vi "MergeFileAutoConfigMARLIN.vi"(4 "error in (no error)":errorcluster, 6 "test num":u32, 7 "ProjetIN":string) -> (0 "error out":errorcluster, 2 "MergeFileConfigOUT":T1, 3 "ProjetOUT":string)   [LabVIEW 2017]
uses:
  DefDeType/MergeFileConfig.ctl
  DefDeType/WhichPath.ctl
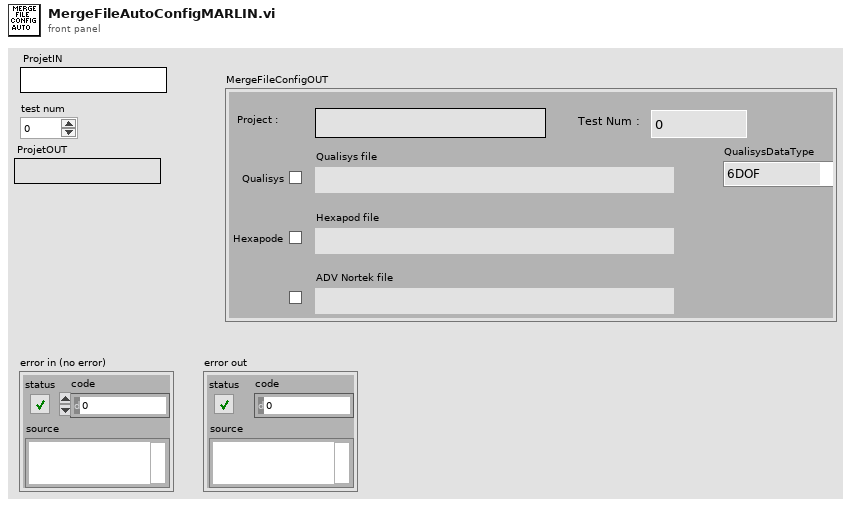
[diagram p1: front panel]
types:
  T1 = typedef "MergeFileConfig.ctl" = cluster{"Test Num : ":u32, "Project :":string, "Qualisys file":path, "Hexapod file":path, "ADV Nortek file":path, "QualisysDataType":enum16{"6DOF", "3DTracking", "6DOF + 3D"}, "Qualisys":bool, "Hexapode":bool, "ADV Nortek":bool}
  T2 = typedef "WhichPath.ctl" = enum16{"DossierProjet", "Config", "Meas", "MeasSuitCase", "MeasOnBoard", "MeasQualisys", "MeasTDMS", "MeasHexapode", "MeasNortek", "Fig", "Res", "MeasUSB"}
  T3 = typedef "WhichPath.ctl" = enum16{"DossierProjet", "Config", "Meas", "MeasPCI", "MeasCRIO1", "MeasCRIO2", "MeasQualisys", "MeasHBM", "MeasTDMS", "Fig", "Res"}
  T4 = typedef "ConfigTotale.ctl" = cluster{"VoltageChannels":T5, "WheastoneBridgeChannels":T6, "Configuration":T7}
  T5 = typedef "VoltageChannels.ctl" = cluster{"ChannelNames":string[], "Sensitivity(Unit/V)":dbl[], "AutoZero":bool[], "ChannelUnits":string[], "Offsets(Units)":dbl[], "Graph Num":u8[]}
  T6 = typedef "WBridgeChannels.ctl" = cluster{"ChannelNames":string[], "Sensitivity(Unit/V)":dbl[], "AutoZero":bool[], "ChannelUnits":string[], "Offsets(Units)":dbl[], "Graph Num":u8[]}
  T7 = typedef "Configuration.ctl" = cluster{"AcqSamplingRate(Hz)":u32, "AcqTime(s)":u32, "Trigger":bool, "NbVoltageChannels":u32, "NbWBridgeChannels":u32, "Qualisys":bool, "Hexapode":bool, "FinalSamplingRate(Hz)":u32, "QualisysDataType":enum16{"6DOF", "3DTracking", "6DOF + 3D"}, "Nortek":bool, "HBM":bool}
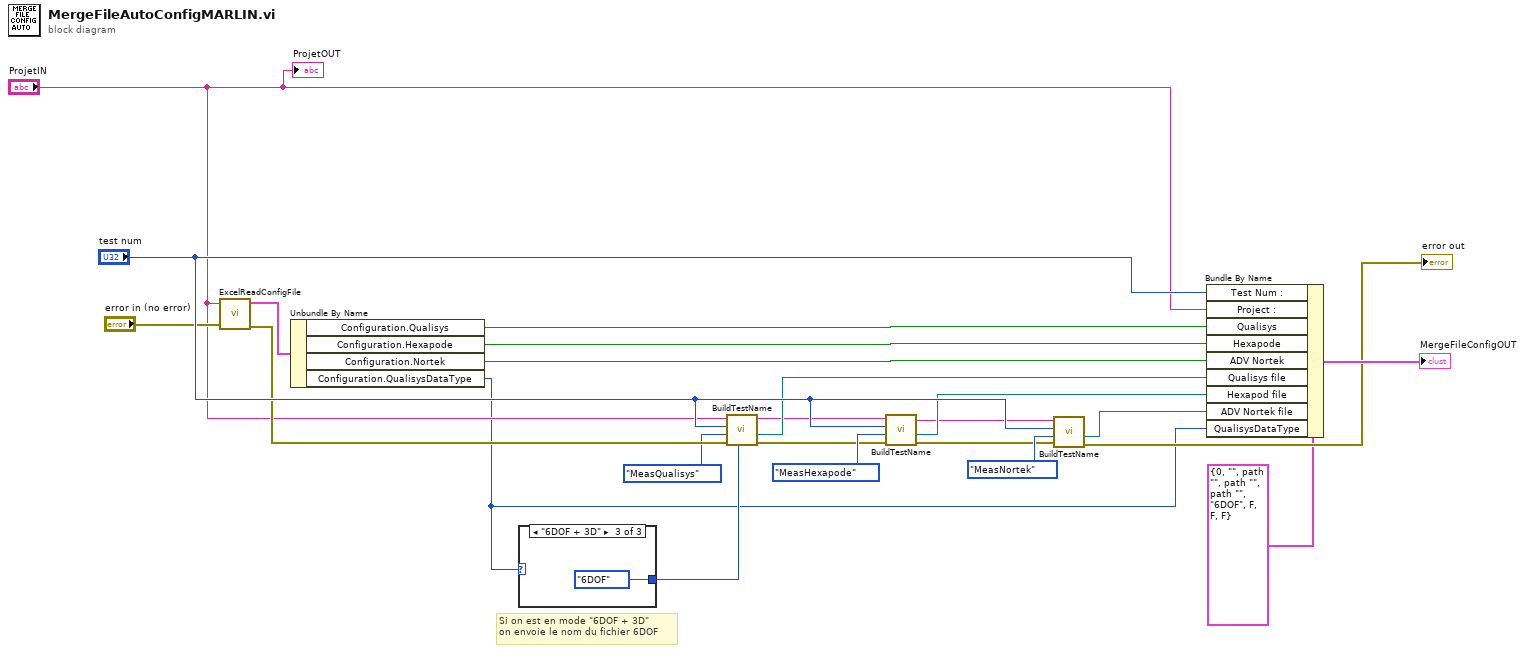
[diagram p0: block diagram]
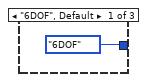
[diagram p2: hidden frame]
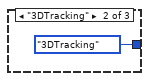
[diagram p3: hidden frame]
diagram:
  # "Si on est en mode \"6DOF + 3D\" \non envoie le nom du fichier 6DOF"
  n1 = call "ExcelReadConfigFile.vi"("NomProjet"="ProjetIN", "error in (no error)"="error in (no error)") -> ("ConfigurationTotale"=w5:T4, "error out"=w20:errorcluster)  [unwired: 3 in]
  n2 = Unbundle By Name(w5) -> ("Configuration.Qualisys"=w6:bool, "Configuration.Hexapode"=w7:bool, "Configuration.Nortek"=w8:bool, "Configuration.QualisysDataType"=w1:enum16{"6DOF", "3DTracking", "6DOF + 3D"})
  n3 = case shown="\"6DOF + 3D\"" w1 {
    tunnel: [enum16{"6DOF", "3DTracking"}."6DOF" ("QualisysDataType") enum16{"6DOF", "3DTracking"}."3DTracking" ("QualisysDataType") enum16{"6DOF", "3DTracking"}."6DOF" ("QualisysDataType")] -> w2
    frame "6DOF", Default {
    }
    frame "3DTracking" {
    }
    frame "6DOF + 3D" {
    }
  }
  n4 = call "BuildTestName.vi"("QualisysDataType"=w2, "entrée d'erreur"=w20, "WhichPath?"=WhichPath."MeasQualisys", "NextTestNum"="test num", "NomProjet"="ProjetIN") -> ("sortie d'erreur"=w11:errorcluster, "cheminProchainFichier"=w17:path, "NomProjetOut"=w13:string)  [unwired: 1 out]
  n5 = call "BuildTestName.vi"("entrée d'erreur"=w11, "WhichPath?"=WhichPath."MeasHexapode", "NextTestNum"="test num", "NomProjet"=w13) -> ("sortie d'erreur"=w14:errorcluster, "cheminProchainFichier"=w18:path, "NomProjetOut"=w16:string)  [unwired: 1 in, 1 out]
  n6 = call "BuildTestName.vi"("entrée d'erreur"=w14, "WhichPath?"=WhichPath."MeasNortek", "NextTestNum"="test num", "NomProjet"=w16) -> ("sortie d'erreur"=→"error out":errorcluster, "cheminProchainFichier"=w19:path)  [unwired: 1 in, 2 out]
  n7 = Bundle By Name(cluster=T1 {"Test Num : "=0, "Project :"="", "Qualisys file"=path "", "Hexapod file"=path "", "ADV Nortek file"=path "", "QualisysDataType"=enum."6DOF", "Qualisys"=FALSE, "Hexapode"=FALSE, "ADV Nortek"=FALSE} ("MergeFileConfig 2"), "Test Num :"="test num", "Project :"="ProjetIN", "Qualisys"=w6, "Hexapode"=w7, "ADV Nortek"=w8, "Qualisys file"=w17, "Hexapod file"=w18, "ADV Nortek file"=w19, "QualisysDataType"=w1) -> (→"MergeFileConfigOUT":T1)
  "ProjetOUT" <- "ProjetIN"
